vi "Sub_Honeywell_voltage_to_displacement.vi"(11 "Pin location voltage":dbl[](array[numeric])) -> (3 "Pin location meters":dbl[](array[numeric]))   [LabVIEW 2021]
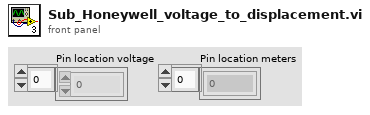
[diagram p1: front panel]
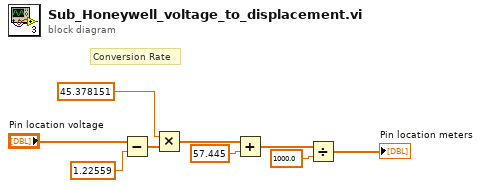
[diagram p0: block diagram]
diagram:
  # "Conversion Rate"
  n1 = Subtract(x="Pin location voltage", y=1.22559) -> (x-y=w4:dbl[])
  n2 = Multiply(x=45.378151, y=w4) -> (x*y=w5:dbl[])
  n3 = Add(x=w5, y=57.445) -> (x+y=w2:dbl[])
  n4 = Divide(x=w2, y=1000.0) -> (x/y=→"Pin location meters":dbl[])
